vi "CLD 10 Step Sequencer with CSV Front Panel.vi"() -> ()   [LabVIEW 2009]
doc: "CLD 10 Exercise"
panel:
  out "Current Step time":dbl
  out "Step 3":bool
  out "Step 2":bool
  out "Step 1":bool
  out "Time Has Elapsed":bool
  out "Elapsed Time (s)":string
  in  "Auto Reset":bool
  in  "Reset Button":bool
  in  "Stop VI":bool
  out "error out":errorcluster
  in  "error in (no error)":errorcluster
  in  "Time Target (s)":dbl
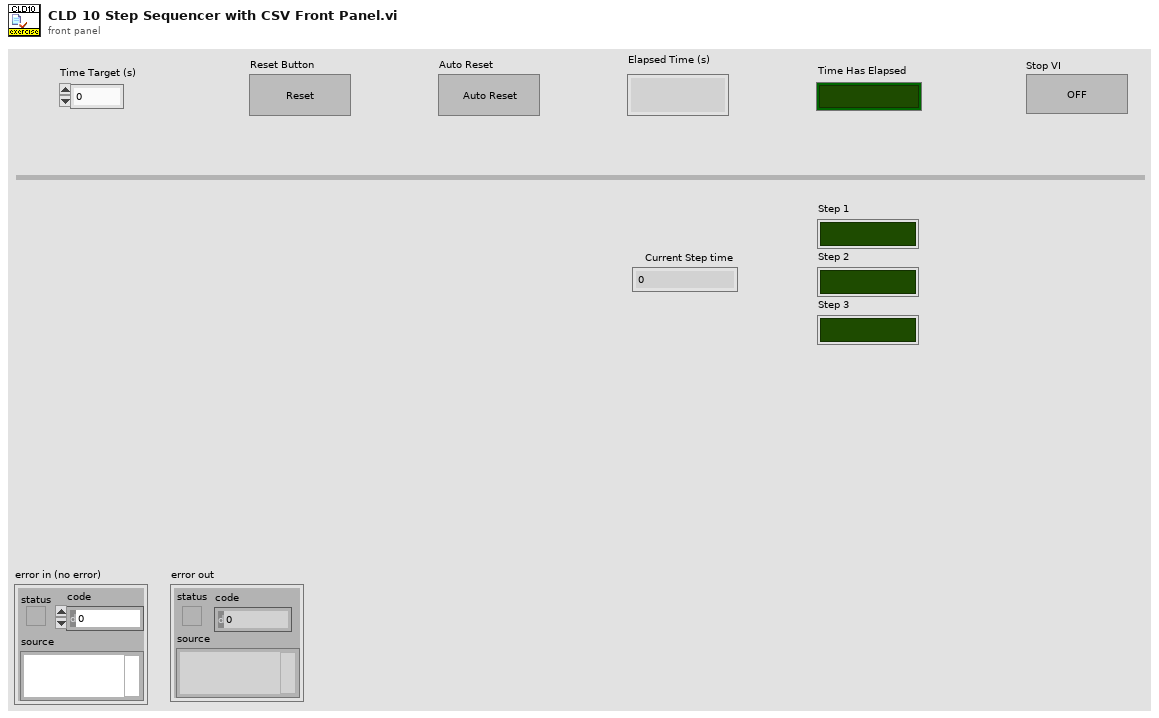
[diagram p1: front panel]
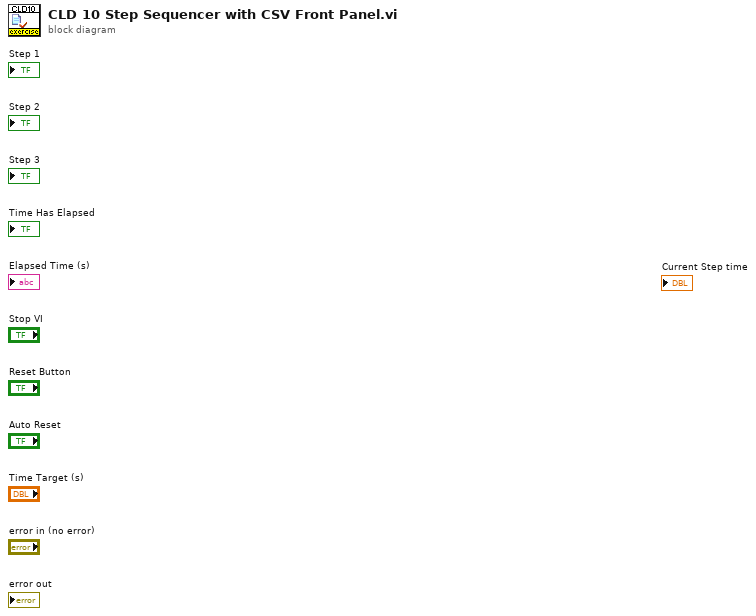
[diagram p0: block diagram]
diagram:
